vi "ControlPid_Motor_Tryhard.vi"() -> ()   [LabVIEW 2025]
uses:
  <vilib>/DAQmx/read.llb/DAQmx Read (Digital 1D Bool 1Chan 1Samp).vi
  <vilib>/DAQmx/create/channels.llb/DAQmx Create Channel (DI-Digital Input).vi
  <vilib>/DAQmx/miscellaneous.llb/DAQmx Fill In Error Info.vi
  <vilib>/addons/control/pid/pid.llb/PID (DBL).vi
  <vilib>/Instr/_visa.llb/VISA Configure Serial Port (Instr).vi
  <vilib>/addons/control/pid/NI_PID_pid.lvlib
panel:
  in  "stop 2":bool
  out "resulting string":string
  out "read buffer":string
  in  "baud rate 115200":u32=9600
  in  "VISA resource name":refnum<visa-resource-name>
  in  "stop":bool
  in  "SetPoint en grados":dbl
  in  "Kp":dbl
  in  "Ki":dbl
  in  "Kd":dbl
  out "Control Output":dbl format="%.2f"
  out "PWM":dbl
  out "Contador de pulsos":dbl
  out "Grados Actuales":dbl
  out "Error":dbl
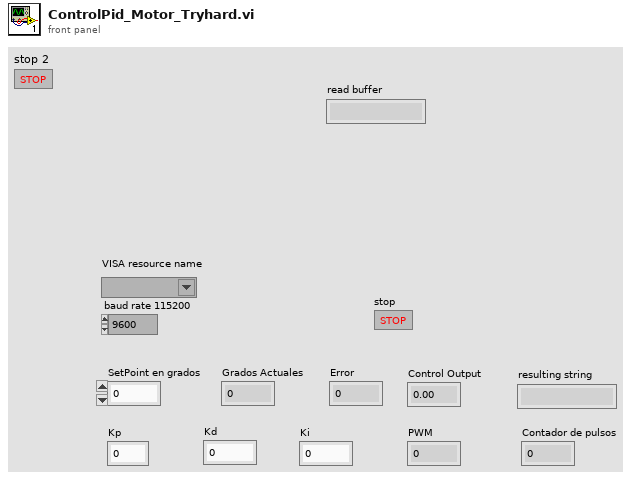
[diagram p1: front panel]
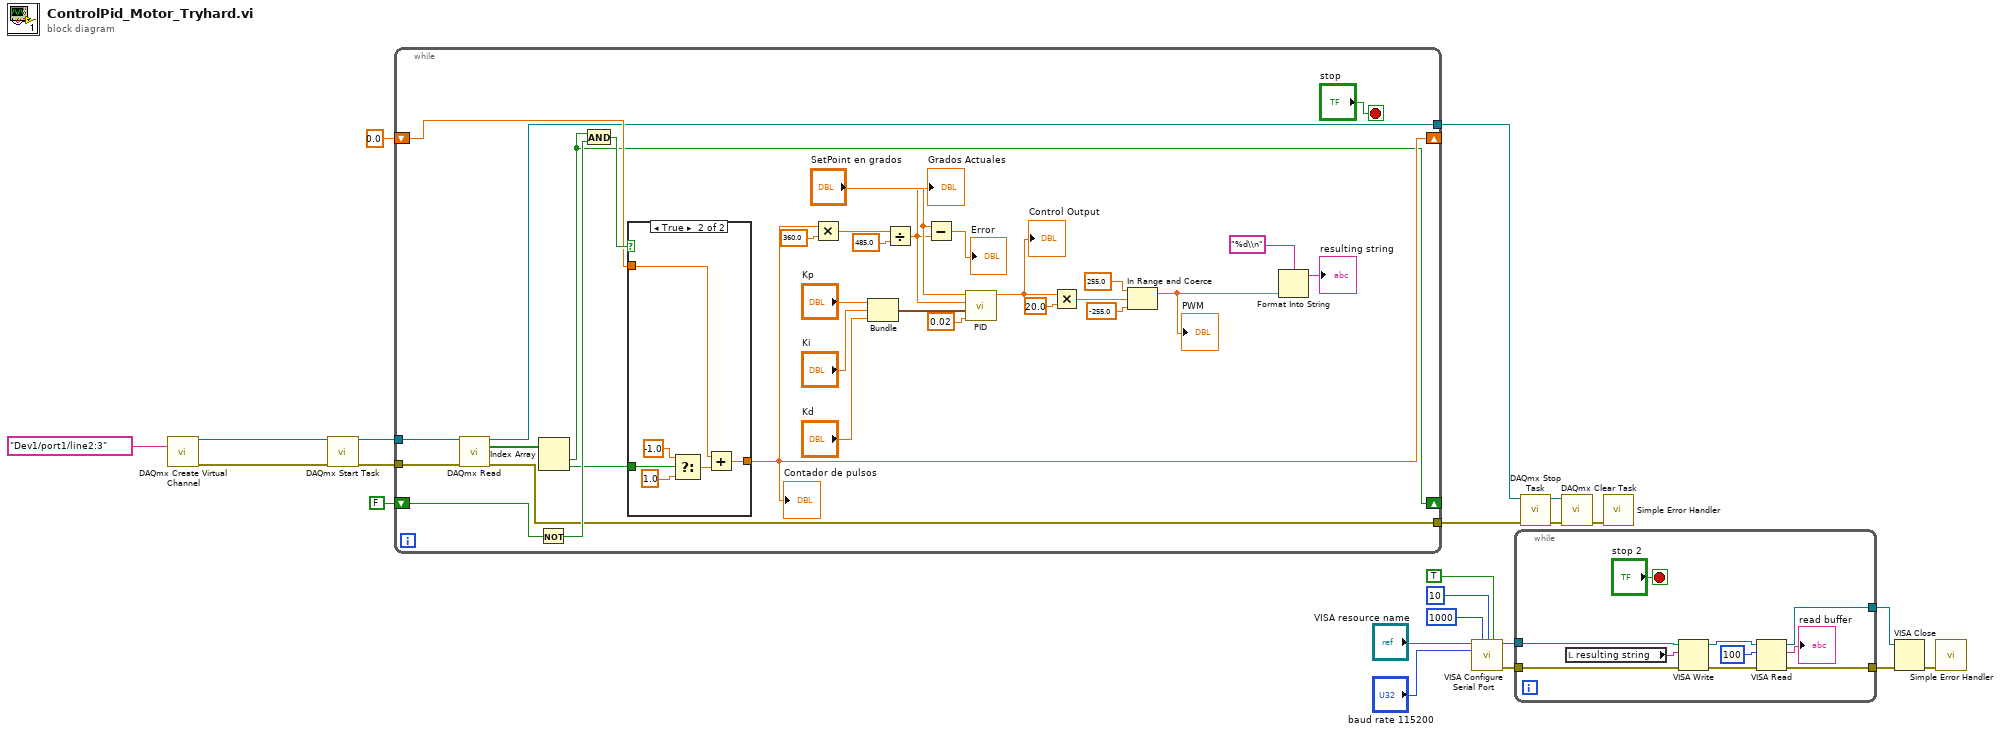
[diagram p0: block diagram]
diagram:
  n1 = call-poly <vilib>:"DAQmx Create Virtual Channel.vi"("lines"=tag "Dev1/port1/line2:3") -> ("task out"=w17:refnum<k21>, "error out"=w16:errorcluster)  [unwired: 13 in]
  n2 = call <vilib>:"DAQmx Start Task.vi"("task/channels in"=w17, "error in"=w16) -> ("task out"=w15:refnum<k21>, "error out"=w14:errorcluster)  [unwired: 12 in]
  n3 = while {
    shift-right: [w37] -> _
    shift-left: 0.0 -> [w41]
    shift-right: [w28] -> _
    shift-left: FALSE -> [w42]
    tunnel: w15 -> [w35]
    tunnel: w14 -> [w36]
    tunnel: [w34] -> w11
    tunnel: [w33] -> w10
    stop <- "stop" stop-if-true
    n4 = call-poly <vilib>:"DAQmx Read.vi"("task/channels in"=w35, "error in"=w36) -> ("task out"=w34:refnum<k21>, "data"=w29:bool[], "error out"=w33:errorcluster)  [unwired: 11 in]
    n5 = Not(x=w42) -> (.not. x?=w54:bool)
    n6 = Index Array(array=w29) -> (element #1=w28:bool, element #2=w27:bool)  [unwired: 2 in]
    n7 = And(x=w28, y=w54) -> (x .and. y?=w53:bool)
    n8 = case shown="True" w53 {
      tunnel: [w55 w58] -> w37
      tunnel: w27 -> [_ w57]
      tunnel: w41 -> [w55 w56]
      frame False {
      }
      frame True {
        n9 = Select(t=-1.0, s=w57, f=1.0) -> (s? t:f=w59:dbl)
        n10 = Add(x=w56, y=w59) -> (x+y=w58:dbl)
      }
    }
    "Contador de pulsos" <- w37
    n11 = Multiply(x=w37, y=360.0) -> (x*y=w39:dbl)
    n12 = Bundle("Kp"="Kp", "Ki"="Ki", "Kd"="Kd") -> (w49:cluster{"Kp":dbl, "Ki":dbl, "Kd":dbl})  [unwired: 1 in]
    n13 = Divide(x=w39, y=485.0) -> (x/y=w30:dbl)
    "Grados Actuales" <- w30
    n14 = Subtract(x="SetPoint en grados", y=w30) -> (x-y=→"Error":dbl)
    n15 = call-poly <vilib>:"PID.vi"("dt (s)"=0.02, "PID gains"=w49, "process variable"=w30, "setpoint"="SetPoint en grados") -> ("output"=w48:dbl)  [unwired: 6 in, 1 out]
    "Control Output" <- w48
    n16 = Multiply(x=w48, y=20.0) -> (x*y=w44:dbl)
    n17 = In Range and Coerce(upper limit=255.0, x=w44, lower limit=-255.0) -> (coerced(x)=w25:dbl)  [unwired: 1 out]
    "PWM" <- w25
    n18 = Format Into String(format string="%d\\n", w25) -> (resulting string=→"resulting string":string)  [unwired: 2 in, 1 out]
  }
  n19 = call-poly "VISA Configure Serial Port"("VISA resource name"="VISA resource name", "timeout (10sec)"=u32 1000, "termination char\n(0xA = '\\n' = LF)"=u8 10 ("termination char\n(0xA = '\\n' = LF)"), "Enable Termination\nChar (T)"=TRUE ("Enable Termination\nChar (T)"), "baud rate (9600)"="baud rate 115200") -> ("VISA resource name out"=w4:refnum<visa-resource-name>, "error out"=w3:errorcluster)  [unwired: 9 in]
  n20 = while {
    tunnel: w4 -> [w67]
    tunnel: w3 -> [w66]
    tunnel: [w65] -> w2
    tunnel: [w64] -> w1
    stop <- "stop 2" stop-if-true
    n21 = local read "resulting string"() -> (w63:string)
    n22 = VISA Write(VISA resource name=w67, write buffer=w63, error in (no error)=w66) -> (VISA resource name out=w69:refnum<visa-resource-name>, error out=w70:errorcluster)  [unwired: 1 out]
    n23 = VISA Read(VISA resource name=w69, byte count=u32 100, error in (no error)=w70) -> (VISA resource name out=w65:refnum<visa-resource-name>, read buffer=→"read buffer":string, error out=w64:errorcluster)  [unwired: 1 out]
  }
  n24 = call <vilib>:"DAQmx Stop Task.vi"("task/channels in"=w11, "error in"=w10) -> ("task out"=w12:refnum<k21>, "error out"=w13:errorcluster)  [unwired: 12 in]
  n25 = call <vilib>:"DAQmx Clear Task.vi"("task in"=w12, "error in"=w13) -> ("error out"=w8:errorcluster)  [unwired: 13 in]
  n26 = call <vilib>:"Simple Error Handler.vi"("error in (no error)"=w8) -> ()  [unwired: 4 in, 5 out]
  n27 = VISA Close(VISA resource name=w2, error in (no error)=w1) -> (error out=w9:errorcluster)
  n28 = call <vilib>:"Simple Error Handler.vi"("error in (no error)"=w9) -> ()  [unwired: 4 in, 5 out]
